vi "Check Action.vi"(6 "HRS Time":dbl, 7 "Values In":dbl[](array[numeric]), 8 "error in (no error)":errorcluster, 11 "Valve in":refnum<class "BangBangControl.lvclass">) -> (0 "error out":errorcluster, 2 "Actions":T1[](array[typedef]), 3 "Valve out":refnum<class "BangBangControl.lvclass">, 5 "Values":dbl[](array[numeric]))   [LabVIEW 2020, in "VolatusControl.lvlib" / "BangBangControl.lvclass"]
uses:
  BangBangControl.lvclass
  Control Action.ctl
  BangBangControl.lvclass/BangBangControl.ctl
  State.ctl
  Volatus/MessageQ/MessageQ.lvclass
  VolatusControl.lvlib
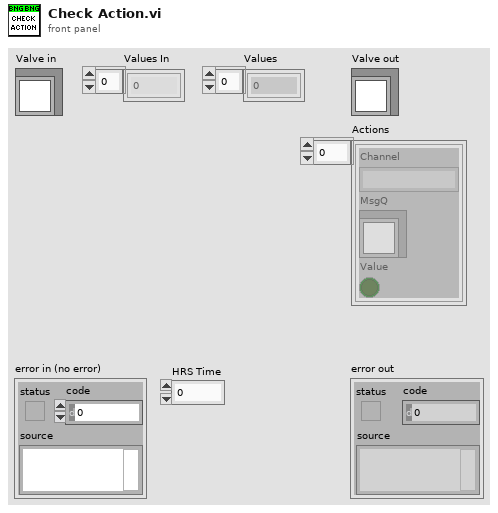
[diagram p1: front panel]
types:
  T1 = typedef "VolatusControl.lvlib/Control Action.ctl" = cluster{"Channel":string, "MsgQ":refnum<class "MessageQ.lvclass">, "Value":bool}
  T2 = typedef "VolatusControl.lvlib/BangBangControl.lvclass/State.ctl" = enum16{"Idle", "RampUp", "RampDown", "Hold", "Disable", "Enable"}
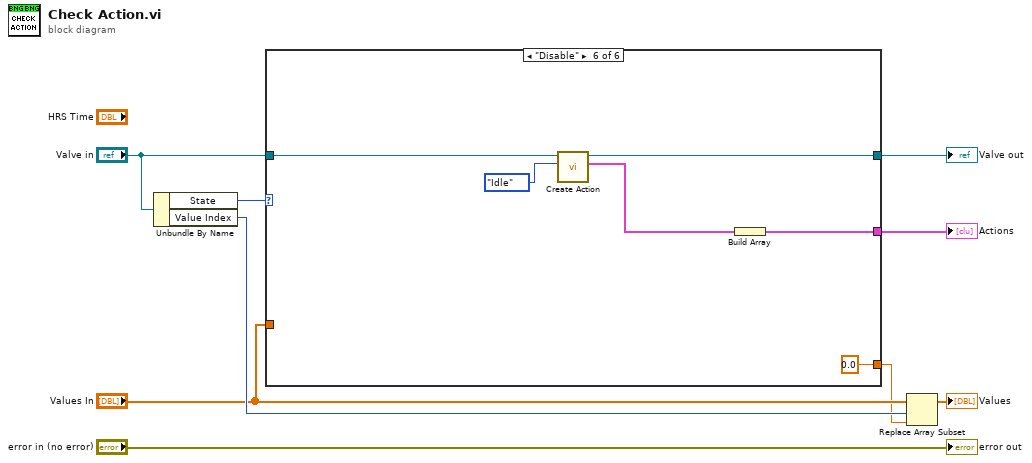
[diagram p0: block diagram]
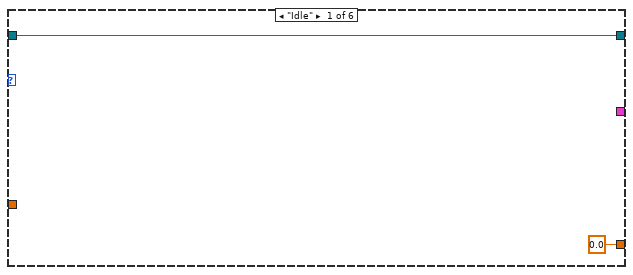
[diagram p2: hidden frame]
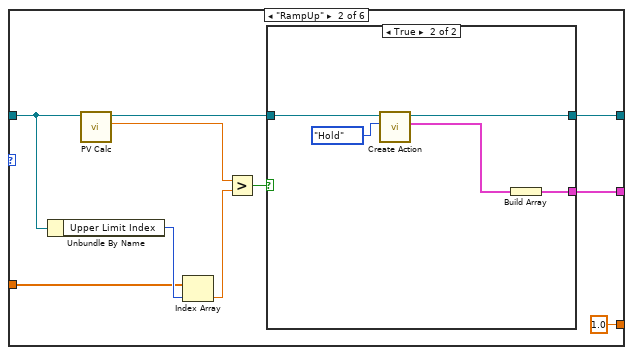
[diagram p3: hidden frame]
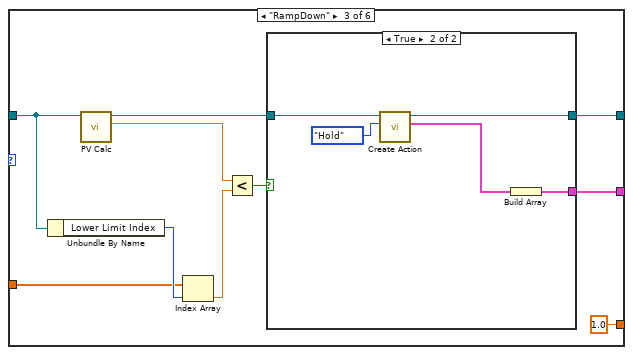
[diagram p5: hidden frame]
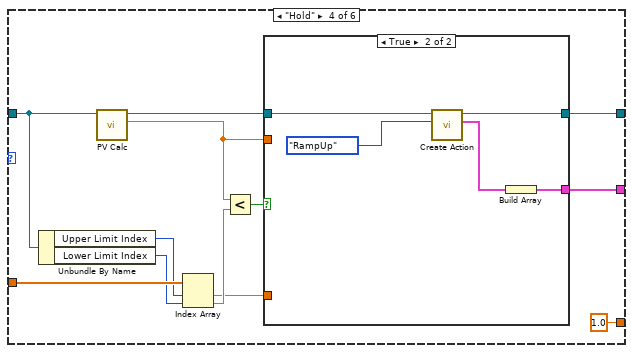
[diagram p7: hidden frame]
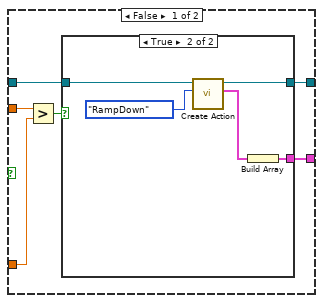
[diagram p8: hidden frame]
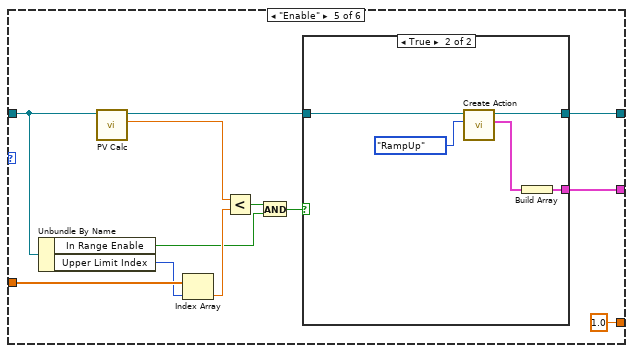
[diagram p10: hidden frame]
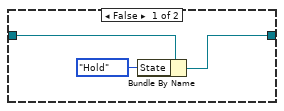
[diagram p11: hidden frame]
diagram:
  n1 = Unbundle By Name("Valve in") -> ("State"=w6:T2, "Value Index"=w7:i32)
  n2 = case shown="\"Disable\"" w6 {
    tunnel: "Values In" -> [_ w19 w35 w53 w82 _]
    tunnel: [0.0 1.0 1.0 1.0 1.0 0.0] -> w4
    tunnel: "Valve in" -> [w10 w21 w37 w54 w83 w97]
    tunnel: [w10 w13 w29 w47 w78 w96] -> w2
    tunnel: [_ w12 w28 w46 w77 w93] -> w1
    frame "Idle" {
    }
    frame "RampUp" {
      n3 = Unbundle By Name(w21) -> ("Upper Limit Index"=w20:i32)
      n4 = call "PV Calc.vi"("BangBangControl in"=w21) -> ("PV"=w15:dbl, "BangBangControl out"=w17:refnum<class "BangBangControl.lvclass">)  [unwired: 8 in, 1 out]
      n5 = Index Array(array=w19, index=w20) -> (element=w16:dbl)
      n6 = Greater?(x=w15, y=w16) -> (0:w14:bool)
      n7 = case shown="True" w14 {
        tunnel: w17 -> [w22 w27]
        tunnel: [w22 w26] -> w13
        tunnel: [_ w23] -> w12
        frame False {
        }
        frame True {
          n8 = call "Create Action.vi"("State"=State."Hold", "BangBangControl in"=w27) -> ("Action"=w24:T1, "BangBangControl out"=w26:refnum<class "BangBangControl.lvclass">)  [unwired: 7 in, 1 out]
          n9 = Build Array(w24) -> (w23:T1[])
        }
      }
    }
    frame "RampDown" {
      n10 = Unbundle By Name(w37) -> ("Lower Limit Index"=w36:i32)
      n11 = call "PV Calc.vi"("BangBangControl in"=w37) -> ("PV"=w31:dbl, "BangBangControl out"=w33:refnum<class "BangBangControl.lvclass">)  [unwired: 8 in, 1 out]
      n12 = Index Array(array=w35, index=w36) -> (element=w32:dbl)
      n13 = Less?(x=w31, y=w32) -> (x < y?=w30:bool)
      n14 = case shown="True" w30 {
        tunnel: w33 -> [w38 w43]
        tunnel: [w38 w42] -> w29
        tunnel: [_ w39] -> w28
        frame False {
        }
        frame True {
          n15 = call "Create Action.vi"("State"=State."Hold", "BangBangControl in"=w43) -> ("Action"=w40:T1, "BangBangControl out"=w42:refnum<class "BangBangControl.lvclass">)  [unwired: 7 in, 1 out]
          n16 = Build Array(w40) -> (w39:T1[])
        }
      }
    }
    frame "Hold" {
      n17 = Unbundle By Name(w54) -> ("Upper Limit Index"=w51:i32, "Lower Limit Index"=w52:i32)
      n18 = call "PV Calc.vi"("BangBangControl in"=w54) -> ("PV"=w44:dbl, "BangBangControl out"=w48:refnum<class "BangBangControl.lvclass">)  [unwired: 8 in, 1 out]
      n19 = Index Array(array=w53, index #1=w51, index #2=w52) -> (element #1=w45:dbl, element #2=w50:dbl)
      n20 = Less?(x=w44, y=w50) -> (x < y?=w49:bool)
      n21 = case shown="True" w49 {
        tunnel: w48 -> [w59 w70]
        tunnel: [w57 w72] -> w47
        tunnel: [w56 w68] -> w46
        tunnel: w45 -> [w60 _]
        tunnel: w44 -> [w61 _]
        frame False {
          n22 = Greater?(x=w61, y=w60) -> (0:w58:bool)
          n23 = case shown="True" w58 {
            tunnel: w59 -> [w62 w65]
            tunnel: [w62 w67] -> w57
            tunnel: [_ w63] -> w56
            frame False {
            }
            frame True {
              n24 = call "Create Action.vi"("State"=State."RampDown", "BangBangControl in"=w65) -> ("Action"=w66:T1, "BangBangControl out"=w67:refnum<class "BangBangControl.lvclass">)  [unwired: 7 in, 1 out]
              n25 = Build Array(w66) -> (w63:T1[])
            }
          }
        }
        frame True {
          n26 = call "Create Action.vi"("State"=State."RampUp", "BangBangControl in"=w70) -> ("Action"=w71:T1, "BangBangControl out"=w72:refnum<class "BangBangControl.lvclass">)  [unwired: 7 in, 1 out]
          n27 = Build Array(w71) -> (w68:T1[])
        }
      }
    }
    frame "Enable" {
      n28 = Unbundle By Name(w83) -> ("In Range Enable"=w73:bool, "Upper Limit Index"=w81:i32)
      n29 = call "PV Calc.vi"("BangBangControl in"=w83) -> ("PV"=w76:dbl, "BangBangControl out"=w79:refnum<class "BangBangControl.lvclass">)  [unwired: 8 in, 1 out]
      n30 = Index Array(array=w82, index=w81) -> (element=w75:dbl)
      n31 = Less?(x=w76, y=w75) -> (x < y?=w80:bool)
      n32 = And(x=w80, y=w73) -> (x .and. y?=w74:bool)
      n33 = case shown="True" w74 {
        tunnel: w79 -> [w87 w90]
        tunnel: [w86 w92] -> w78
        tunnel: [_ w88] -> w77
        frame False {
          n34 = Bundle By Name(cluster=w87, "State"=State."Hold") -> (w86:refnum<class "BangBangControl.lvclass">)
        }
        frame True {
          n35 = call "Create Action.vi"("State"=State."RampUp", "BangBangControl in"=w90) -> ("Action"=w91:T1, "BangBangControl out"=w92:refnum<class "BangBangControl.lvclass">)  [unwired: 7 in, 1 out]
          n36 = Build Array(w91) -> (w88:T1[])
        }
      }
    }
    frame "Disable" {
      n37 = call "Create Action.vi"("State"=State."Idle", "BangBangControl in"=w97) -> ("Action"=w94:T1, "BangBangControl out"=w96:refnum<class "BangBangControl.lvclass">)  [unwired: 7 in, 1 out]
      n38 = Build Array(w94) -> (w93:T1[])
    }
  }
  "Valve out" <- w2
  "Actions" <- w1
  n39 = Replace Array Subset(array="Values In", new element=w4, index=w7) -> (→"Values":dbl[])
  "error out" <- "error in (no error)"
